vi "Is Recieve Ready.vi"(8 "error in (no error)":errorcluster, 11 "RP Lockin in":refnum<class "RP Transceiver.lvclass">) -> (0 "error out":errorcluster, 2 "Recieve Ready":bool, 3 "RP Lockin out":refnum<class "RP Transceiver.lvclass">)   [LabVIEW 2015, in "RP Transceiver.lvclass"]
uses:
  RP Transceiver.lvclass
  RP Transceiver.lvclass/RP Transceiver.ctl
  RP Communicator/RP Communicator.lvclass
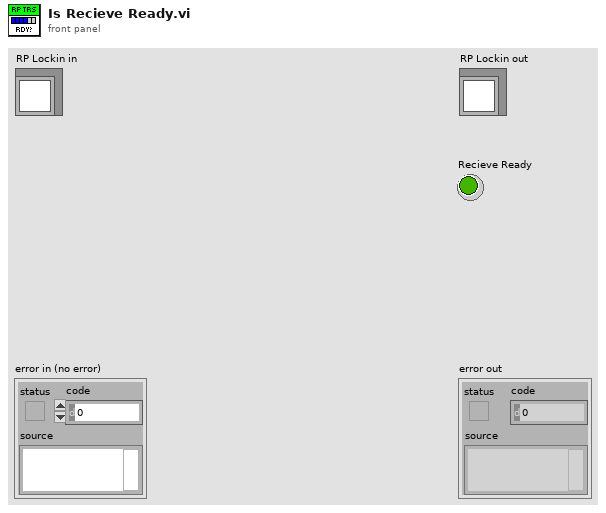
[diagram p1: front panel]
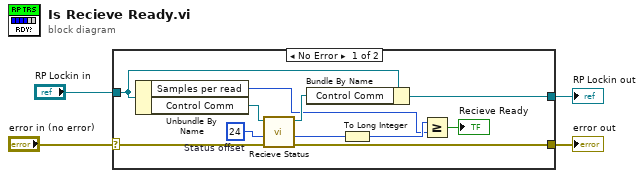
[diagram p0: block diagram]
diagram:
  n1 = case shown="No Error" "error in (no error)" {
    selector: "error in (no error)" -> [w7 w17]
    tunnel: [w6 w17] -> w3
    tunnel: [w9 w16] -> w1
    tunnel: "RP Lockin in" -> [w15 w16]
    frame No Error {
      w13 = u64 24  # Status offset
      n2 = Unbundle By Name(w15) -> ("Samples per read"=w5:i32, "Control Comm"=w14:refnum<class "RP Communicator.lvclass">)
      n3 = call-dynamic "Recieve Status.vi"("error in (no error)"=w7, "Status offset"=w13, "RP Communicator in"=w14) -> ("error out"=w6:errorcluster, "Status response"=w11:u32, "RP Communicator out"=w8:refnum<class "RP Communicator.lvclass">)  [unwired: 6 in]
      n4 = Bundle By Name(cluster=w15, "Control Comm"=w8) -> (w9:refnum<class "RP Transceiver.lvclass">)
      n5 = To Long Integer(number=w11) -> (32bit integer=w12:i32)
      n6 = Greater Or Equal?(x=w12, y=w5) -> (x >= y?=→"Recieve Ready":bool)
    }
    frame Error {
    }
  }
  "error out" <- w3
  "RP Lockin out" <- w1
